vi "CreateFolderWithDate.vi"() -> ()   [LabVIEW 2018]
panel:
  in  "Subfolder":string="Sample1"
  in  "Output Path":path=path "F:/Data_Min"
  in  "Folder Name":string="Test"
  in  "File Name":string="Pos1"
  # "Path/Folders"
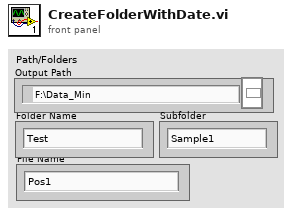
[diagram p1: front panel]
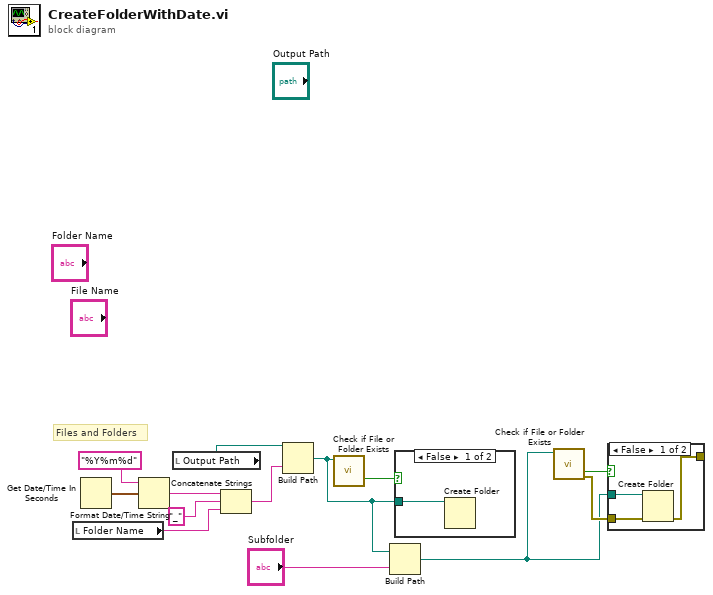
[diagram p0: block diagram]
diagram:
  # "Files and Folders"
  n1 = local read "Folder Name"() -> (w5:string)
  n2 = Get Date/Time In Seconds() -> (seconds since 1Jan1904=w10:timestamp)
  n3 = Format Date/Time String(time format string (%c)="%Y%m%d", seconds (now)=w10) -> (date/time string=w9:string)  [unwired: 1 in]
  n4 = local read "Output Path"() -> (w6:path)
  n5 = Concatenate Strings(w9, "_", w5) -> (w8:string)
  n6 = Build Path(base path=w6, name or relative path=w8) -> (appended path=w2:path)
  n7 = call <vilib>:"Check if File or Folder Exists.vi"("path"=w2) -> ("file or folder exists?"=w13:bool)  [unwired: 8 in, 2 out]
  n8 = Build Path(base path=w2, name or relative path="Subfolder") -> (appended path=w1:path)
  n9 = case shown="False" w13 {
    tunnel: w2 -> [w14 _]
    frame False {
      n10 = Create Folder(path (use dialog)=w14) -> ()  [unwired: 2 in, 3 out]
    }
    frame True {
    }
  }
  n11 = call <vilib>:"Check if File or Folder Exists.vi"("path"=w1) -> ("error out"=w4:errorcluster, "file or folder exists?"=w12:bool)  [unwired: 8 in, 1 out]
  n12 = case shown="False" w12 {
    tunnel: w1 -> [w17 _]
    tunnel: w4 -> [w16 w18]
    tunnel: [w15 w18] -> _
    frame False {
      n13 = Create Folder(path (use dialog)=w17, error in=w16) -> (error out=w15:errorcluster)  [unwired: 1 in, 2 out]
    }
    frame True {
    }
  }
